vi "ReadData.vi"(10 "samples per read":i32, 11 "path":path) -> (1 "runtime (ms)":dbl format="%#_6f")   [LabVIEW 2016]
uses:
  <vilib>/Analysis/Matrix/Numeric/Conversions/Array To Matrix - RA2.vi
  <vilib>/Analysis/Matrix/NI_Matrix.lvlib
panel:
  in  "Tab Control":enum32{"Page 1", "Page 2"}(tab)
  out "file size (in samples)":dbl format="%#_6f"
  out "Percent Done":dbl
  out "Counter":i32
  out "start time (ms)":u32
  out "stop time (ms)":u32
  in  "byte order":T1(ring)
  out "Complex Out":cdb[][](array[numeric])
  # "Setup Input"
  # "Runtime Output"
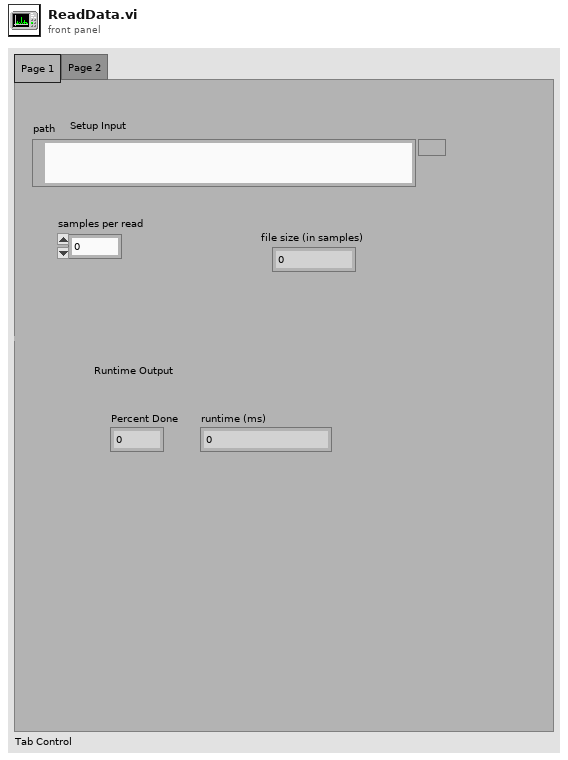
[diagram p1: front panel]
types:
  T1 = enum16{"big-endian, network order", "native, host order", "little-endian"}
  T2 = typedef "NI_Matrix.lvlib/RealMatrix.ctl" = dbl[][]
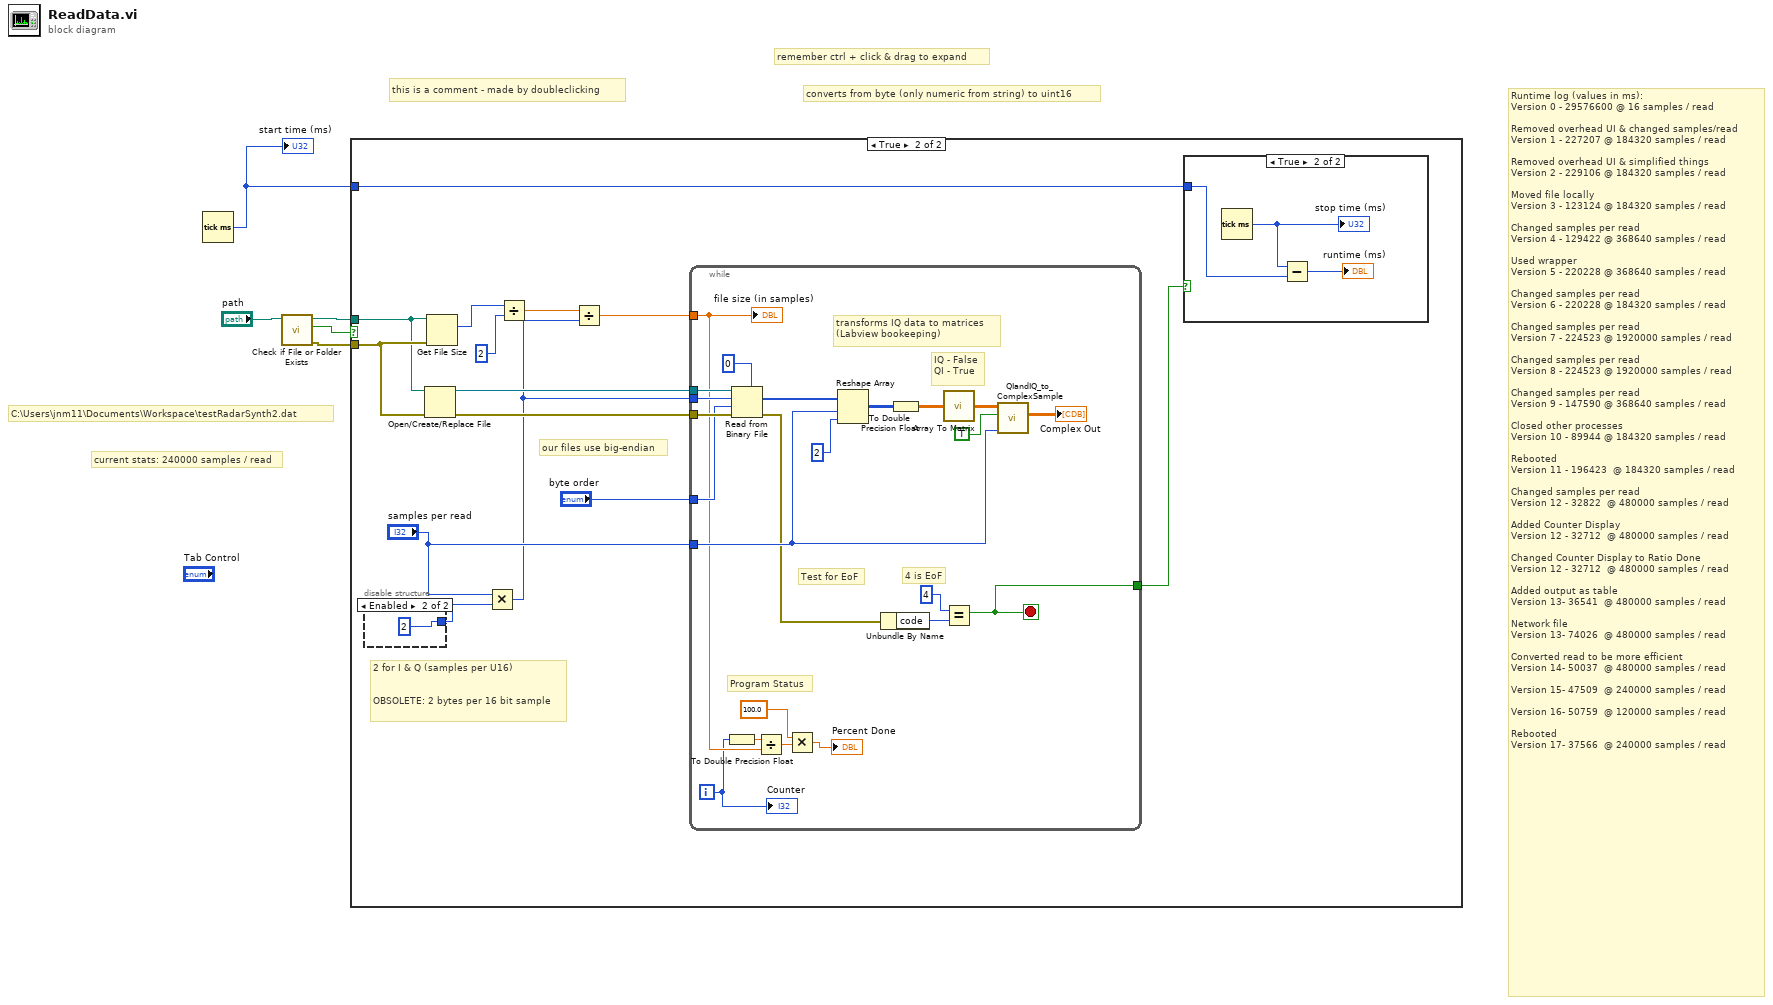
[diagram p0: block diagram]
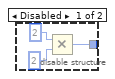
[diagram p3: hidden frame]
diagram:
  # "current stats: 240000 samples / read"
  # "C:\\Users\\jnm11\\Documents\\Workspace\\testRadarSynth2.dat"
  # "Runtime log (values in ms):\nVersion 0 - 29576600 @ 16 samples / read\n\nRemoved overhead UI & changed samples/read\nVersion 1 - 227207 @ 184320 samples / read\n\nRemoved overhead UI & simplified things \nVersion 2 - 229106 @ 184320 samples / read\n\nMoved file locally\nVersion 3 - 123124 @ 184320 samples / read\n\nChanged samples per read\nVersion 4 - 129422 @ 368640 samples / read\n\nUsed wrapper\nVersion 5 - 220228 @ 368640 samples / read\n\nChanged samples per read\nVersion 6 - 220228 @ 184320 samples / read\n\nChanged samples per read\nVersion 7 - 224523 @ 1920000 samples / read\n\nChanged samples per read\nVersion 8 - 224523 @ 1920000 samples / read\n\nChanged samples per read\nVersion 9 - 147590 @ 368640 samples / read\n\nClosed other processes\nVersion 10 - 89944 @ 184320 samples / read\n\nRebooted\nVersion 11 - 196423  @ 184320 samples / read\n\nChanged samples per read\nVersion 12 - 32822  @ 480000 samples / read\n\nAdded Counter Display\nVersion 12 - 32712  @ 480000 samples / read\n\nChanged Counter Display to Ratio Done\nVersion 12 - 32712  @ 480000 samples / read\n\nAdded output as table\nVersion 13- 36541  @ 480000 samples / read\n\nNetwork file\nVersion 13- 74026  @ 480000 samples / read\n\nConverted read to be more efficient\nVersion 14- 50037  @ 480000 samples / read\n\nVersion 15- 47509  @ 240000 samples / read\n\nVersion 16- 50759  @ 120000 samples / read\n\nRebooted\nVersion 17- 37566  @ 240000 samples / read"
  # "converts from byte (only numeric from string) to uint16"
  # "remember ctrl + click & drag to expand"
  # "this is a comment - made by doubleclicking"
  n1 = Tick Count (ms)() -> (millisecond timer value=w1:u32)
  "start time (ms)" <- w1
  n2 = call <vilib>:"Check if File or Folder Exists.vi"("path"="path") -> ("error out"=w2:errorcluster, "file or folder exists?"=w3:bool, "dup path"=w4:path)  [unwired: 8 in]
  n3 = case shown="True" w3 {
    tunnel: w4 -> [_ w18]
    tunnel: w2 -> [_ w19]
    tunnel: w1 -> [_ w12]
    frame False {
    }
    frame True {
      # "2 for I & Q (samples per U16)\n\n\nOBSOLETE: 2 bytes per 16 bit sample"
      # "our files use big-endian"
      n4 = disable-structure shown="Enabled" {
        disable-tunnel: [w20 2 ("y")] -> w10
        frame Disabled {
          n5 = Multiply(x=2 ("column N"), y=2 ("column N")) -> (x*y=w20:i32)
        }
        frame Enabled {
        }
      }
      n6 = Open/Create/Replace File(file path (use dialog)=w18, error in=w19) -> (refnum out=w17:refnum<file>, error out=w16:errorcluster)  [unwired: 4 in, 1 out]
      n7 = Get File Size(file=w18, error in=w19) -> (size (in bytes)=w9:i64)  [unwired: 2 out]
      n8 = Multiply(x="samples per read", y=w10) -> (x*y=w6:i32)
      n9 = Divide(x=w9, y=i64 2) -> (x/y=w7:dbl)
      n10 = Divide(x=w7, y=w6) -> (x/y=w13:dbl)
      n11 = while {
        tunnel: w17 -> [w49]
        tunnel: w16 -> [w48]
        tunnel: "byte order" -> [w47]
        tunnel: w6 -> [w46]
        tunnel: "samples per read" -> [w45]
        tunnel: w13 -> [w38]
        tunnel: [w39] -> w11
        i -> [w31]
        stop <- w39 stop-if-true
        # "Test for EoF"
        # "Program Status"
        # "4 is EoF"
        # "transforms IQ data to matrices \n(Labview bookeeping)"
        # "IQ - False\nQI - True"
        n12 = To Double Precision Float(number=w31) -> (double precision float=w33:dbl)
        n13 = Read from Binary File(5:u16 0 ("dimension size"), 8:w48, 9:w47, 10:w46, 11:w49) -> (0:w42:errorcluster, 2:w34:u16[])  [unwired: 1 in, 2 out]
        n14 = Divide(x=w33, y=w38) -> (x/y=w30:dbl)
        n15 = Multiply(x=100.0, y=w30) -> (x*y=→"Percent Done":dbl)
        n16 = Reshape Array(w34, w45, 2 ("dimension size")) -> (w36:u16[][])
        n17 = Unbundle By Name(w42) -> ("code"=w41:i32)
        n18 = To Double Precision Float(number=w36) -> (double precision float=w35:dbl[][])
        n19 = call-poly <vilib>:"Array To Matrix.vi"("Real 2D Array"=w35) -> ("Real Matrix"=w44:T2)
        n20 = Equal?(x=4, y=w41) -> (x = y?=w39:bool)
        n21 = call "QIandIQ_to_ComplexSample.vi"("array size (samples)"=w45, "IQ or QI"=TRUE, "Raw Data (Q,I) - base 10"=w44) -> ("Complex Out"=→"Complex Out":cdb[][])  [unwired: 7 in, 1 out]
        "file size (in samples)" <- w38
        "Counter" <- w31
      }
      n22 = case shown="True" w11 {
        tunnel: w12 -> [_ w24]
        frame False {
        }
        frame True {
          n23 = Tick Count (ms)() -> (millisecond timer value=w26:u32)
          "stop time (ms)" <- w26
          n24 = Subtract(x=w26, y=w24) -> (x-y=→"runtime (ms)":u32)
        }
      }
    }
  }
